vi "2022_day09_Task1_only.vi"() -> ()   [LabVIEW 2021]
panel:
  out "Array 2":bool[][](array[boolean])
  in  "Enum":enum16{"L", "R", "U", "D"}(ring)
  out "Array":cluster{enum16{"L", "R", "U", "D"}, i32}[](array[cluster])
  out "Task 1":i16
  in  "Switch":bool caption="Ex. Data  vs.  User Data"
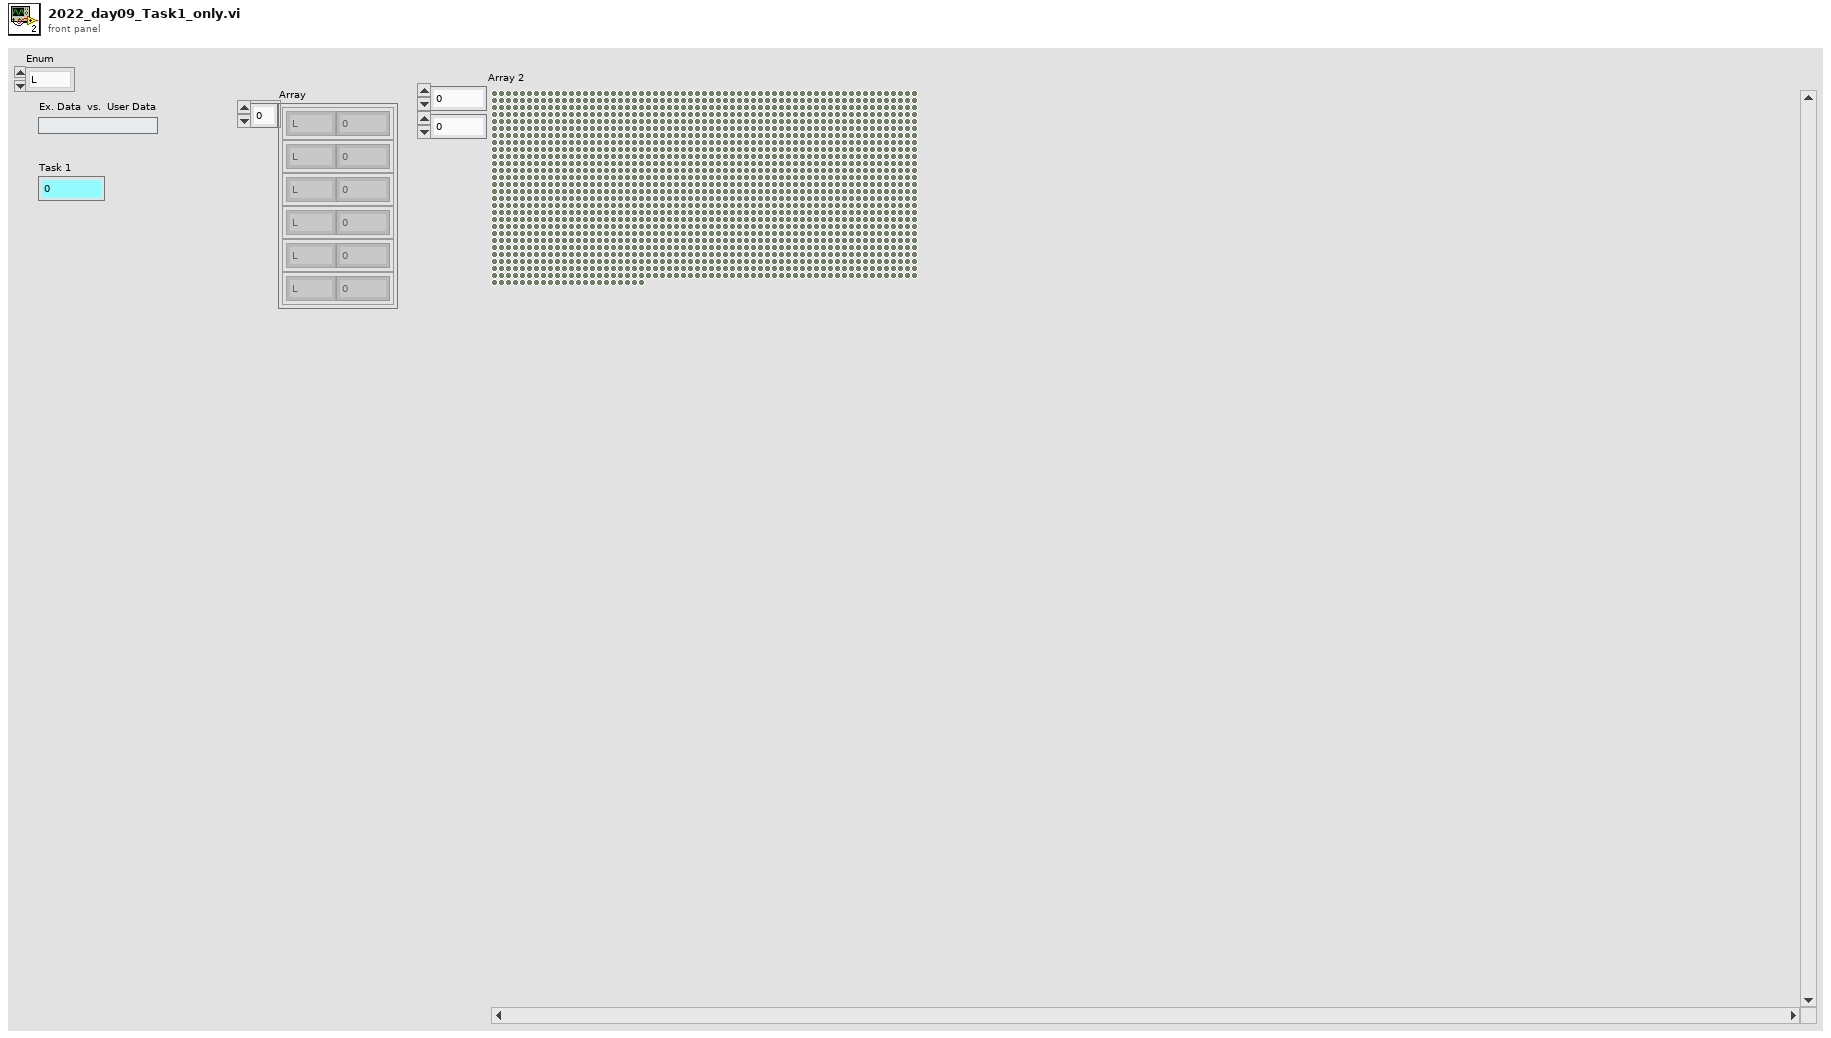
[diagram p1: front panel]
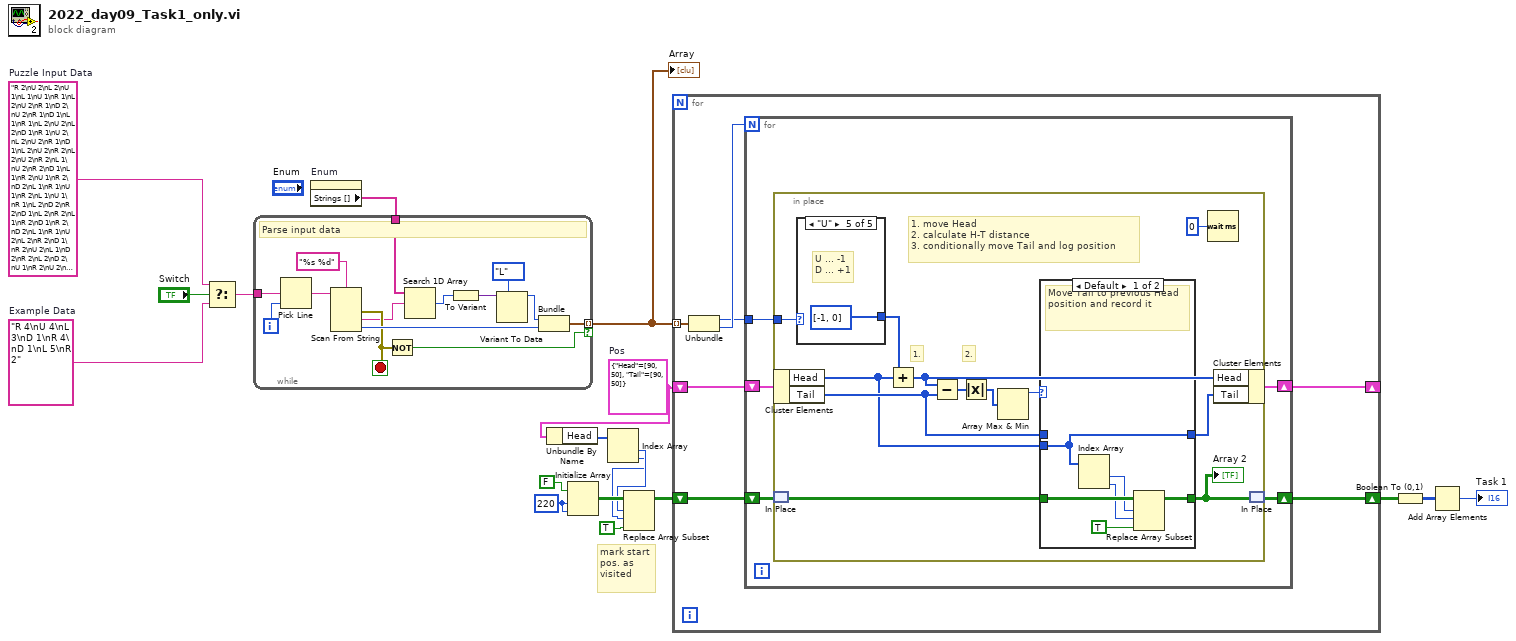
[diagram p0: block diagram]
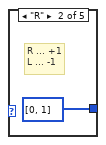
[diagram p4: hidden frame]
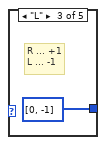
[diagram p5: hidden frame]
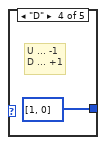
[diagram p6: hidden frame]
diagram:
  w7 = cluster{"Head":i32[], "Tail":i32[]} {"Head"=[90, 50], "Tail"=[90, 50]}  # Pos
  w13 = 220 ("dimension size")
  w17 = "R 2\nU 2\nL 2\nU 1\nL 1\nU 1\nR 1\nL 2\nU 2\nR 1\nD 2\nU 2\nR 1\nD 1\nL 1\nR 1\nL 2\nU 2\nL 2\nD 1\nR 1\nU 2\nL 2\nU 2\nR 1\nD 1\nL 2\nU 2\nR 2\nL 2\nU 2\nR 2\nL 1\nU 2\nR 2\nD 1\nL 1\nR 2\nU 1\nR 2\nD 2\nL 1\nR 1\nU 1\nR 2\nL 1\nU 1\nR 1\nL 2\nD 2\nR 2\nD 1\nL 2\nR 2\nL 1\nR 2\nD 1\nR 2\nD 2\nL 1\nR 1\nU 2\nL 2\nR 2\nD 1\nR 2\nU 2\nL 1\nD 2\nR 2\nL 2\nD 2\nU 1\nR 2\nU 2\nR 2\nD 2\nR 1\nU 2\nD 2\nR 1\nL 1\nR 1\nU 2\nD 2\nR 1\nU 1\nR 1\nL 1\nU 2\nL 2\nD 2\nU 2\nD 2\nR 2\nD 2\nL 1\nU 2\nL 1\nR 1\nD 2\nL 1\nU 1\nD 2\nU 2\nD 2\nR 2\nU 1\nR 1\nU 2\nD 1\nR 2\nD 2\nL 3\nU 1\nD 2\nU 3\nR 3\nL 1\nD 2\nR 1\nD 3\nL 3\nR 1\nD 3\nL 3\nD 1\nR 3\nD 1\nL 1\nD 2\nR 3\nD 1\nU 2\nR 2\nL 1\nD 1\nR 3\nU 2\nL 3\nU 2\nD 2\nR 2\nD 3\nU 1\nD 3\nL 3\nR 2\nL 2\nD 3\nL 2\nU 3\nR 2\nD 1\nR 2\nU 3\nR 3\nU 3\nL 1\nR 3\nD 2\nR 1\nL 3\nR 1\nD 3\nL 3\nD 1\nU 2\nR 3\nU 3\nD 1\nL 2\nR 3\nL 1\nD 2\nL 3\nD 1\nL 3\nD 1\nU 2\nD 3\nR 2\nU 1\nL 3\nR 3\nL 2\nR 1\nL 2\nD 2\nR 3\nU 3\nR 3\nD 2\nU 3\nD 2\nR 3\nD 3\nR 2\nU 1\nL 3\nU 2\nR 2\nL 2\nU 1\nL 3\nD 2\nU 2\nR 1\nL 2\nD 2\nU 3\nR 2\nD 2\nL 3\nU 1\nL 1\nU 2\nR 2\nU 1\nD 2\nU 2\nR 3\nL 1\nU 1\nD 3\nU 4\nL 3\nD 2\nL 3\nU 4\nD 2\nR 4\nL 4\nU 2\nD 3\nU 2\nD 3\nL 3\nU 2\nD 3\nL 1\nU 1\nR 1\nL 4\nR 3\nD 3\nL 2\nU 3\nR 2\nL 1\nU 4\nD 3\nU 1\nL 2\nD 4\nL 1\nR 3\nD 4\nR 1\nL 1\nU 3\nL 3\nD 3\nR 3\nU 1\nL 4\nU 3\nR 3\nL 3\nU 2\nR 3\nL 3\nR 1\nD 3\nR 3\nL 4\nR 3\nD 4\nL 3\nU 2\nR 4\nL 1\nU 1\nR 4\nD 3\nU 1\nR 1\nD 1\nU 3\nR 2\nL 1\nD 1\nL 3\nD 4\nR 4\nU 4\nD 1\nR 3\nD 3\nR 3\nL 4\nR 4\nL 2\nR 2\nD 3\nR 4\nD 2\nU 4\nL 3\nD 1\nR 2\nU 2\nR 3\nD 1\nR 3\nD 1\nL 1\nU 4\nL 2\nU 4\nL 4\nU 3\nR 4\nL 3\nR 3\nL 4\nU 4\nR 4\nD 2\nR 2\nD 3\nU 4\nD 1\nU 1\nD 5\nU 3\nD 5\nU 5\nD 3\nL 3\nU 3\nD 3\nR 1\nD 3\nR 4\nU 4\nD 1\nR 5\nD 5\nR 2\nU 5\nL 2\nU 2\nD 2\nU 4\nR 1\nD 1\nL 2\nR 2\nD 1\nL 5\nR 5\nD 4\nR 5\nL 1\nD 2\nL 3\nU 2\nD 3\nL 1\nR 5\nU 3\nR 1\nD 3\nR 1\nU 1\nR 3\nU 2\nD 5\nL 5\nR 1\nU 3\nL 4\nD 2\nR 1\nD 3\nU 4\nR 3\nL 4\nU 2\nD 3\nU 1\nR 5\nD 3\nL 2\nU 3\nL 5\nU 3\nL 3\nD 5\nL 5\nU 3\nR 2\nD 5\nU 4\nL 5\nU 1\nD 5\nR 3\nD 1\nL 5\nR 2\nD 2\nU 5\nR 1\nD 2\nL 3\nD 2\nL 5\nD 2\nU 5\nL 2\nR 3\nL 3\nD 3\nU 2\nR 5\nL 1\nU 5\nR 5\nL 2\nD 5\nR 3\nL 2\nU 2\nD 3\nR 4\nL 1\nR 3\nD 5\nR 3\nD 4\nR 2\nD 5\nR 3\nL 3\nR 2\nU 2\nL 1\nR 6\nU 6\nL 6\nU 2\nR 6\nD 4\nU 1\nL 1\nR 1\nD 1\nL 6\nD 6\nU 4\nL 6\nD 3\nR 1\nU 1\nD 3\nR 3\nD 5\nU 1\nL 2\nR 6\nU 5\nD 6\nL 6\nR 2\nU 1\nD 1\nL 4\nD 5\nL 6\nU 1\nL 6\nR 5\nU 5\nD 3\nL 5\nR 2\nU 3\nD 1\nL 2\nU 2\nD 1\nL 5\nD 1\nU 5\nR 4\nL 2\nR 5\nD 3\nU 3\nR 2\nU 3\nD 6\nL 5\nR 1\nU 5\nL 1\nR 6\nD 6\nR 6\nL 1\nD 2\nR 5\nL 4\nD 3\nL 5\nR 4\nL 6\nU 1\nL 2\nU 3\nR 4\nD 3\nR 3\nL 1\nD 4\nL 2\nR 5\nD 2\nR 2\nD 5\nU 2\nL 4\nR 4\nU 4\nR 1\nD 3\nL 6\nU 5\nL 5\nD 6\nU 3\nD 6\nR 6\nD 3\nU 6\nL 6\nD 3\nL 6\nR 3\nD 2\nL 4\nD 5\nL 5\nD 2\nL 6\nR 1\nD 1\nL 4\nU 6\nR 1\nL 5\nD 7\nU 2\nR 6\nD 7\nL 2\nR 3\nU 1\nL 3\nR 2\nU 7\nD 7\nU 7\nD 4\nR 2\nL 7\nR 7\nL 5\nR 4\nU 5\nL 5\nU 6\nR 2\nD 3\nL 2\nU 6\nD 5\nR 2\nD 2\nR 5\nU 7\nR 3\nD 1\nL 5\nR 1\nU 3\nD 6\nU 6\nL 7\nU 4\nL 6\nD 1\nL 7\nU 4\nD 7\nL 1\nD 6\nL 2\nR 5\nL 7\nU 3\nD 2\nR 7\nL 2\nU 6\nL 3\nU 6\nL 5\nR 2\nL 7\nD 3\nL 7\nR 1\nL 1\nR 5\nD 6\nL 2\nD 5\nL 4\nD 3\nU 5\nD 1\nR 4\nU 1\nL 2\nR 3\nU 7\nD 6\nU 2\nD 4\nU 5\nD 5\nU 7\nR 2\nD 1\nU 2\nL 2\nU 3\nD 1\nR 4\nD 1\nR 3\nU 1\nR 7\nD 4\nR 3\nD 2\nL 2\nU 4\nL 2\nU 6\nL 4\nD 6\nU 3\nL 1\nU 4\nR 7\nD 6\nL 2\nD 7\nR 4\nU 5\nR 4\nD 5\nR 6\nD 4\nR 4\nU 2\nR 3\nL 7\nR 8\nD 8\nR 5\nU 2\nD 6\nL 2\nR 4\nU 3\nL 1\nR 2\nD 5\nL 1\nD 5\nL 5\nU 1\nR 8\nD 1\nU 1\nL 1\nR 8\nL 3\nR 6\nL 1\nU 3\nR 6\nL 5\nU 2\nL 8\nR 4\nU 4\nR 6\nU 5\nR 1\nL 2\nR 5\nD 1\nU 4\nL 3\nU 3\nR 1\nU 3\nR 8\nL 1\nU 2\nL 7\nD 6\nL 6\nR 4\nD 2\nR 2\nL 8\nD 4\nR 4\nU 4\nL 6\nD 3\nR 7\nD 8\nU 4\nR 4\nU 2\nL 8\nD 5\nL 4\nU 7\nD 8\nU 6\nR 6\nL 5\nD 5\nL 2\nD 1\nR 1\nD 4\nR 5\nL 7\nD 8\nU 2\nD 3\nL 5\nR 4\nL 7\nR 3\nL 1\nD 8\nR 5\nL 8\nR 8\nD 1\nR 4\nD 1\nL 2\nD 5\nL 7\nU 1\nL 4\nR 5\nL 3\nR 9\nD 9\nL 4\nR 6\nL 6\nR 1\nL 3\nR 5\nD 8\nL 1\nU 2\nR 8\nU 7\nD 6\nL 8\nD 1\nL 9\nD 5\nL 1\nD 6\nL 8\nR 2\nL 6\nR 4\nU 1\nR 6\nL 5\nR 5\nL 6\nR 8\nD 5\nL 4\nR 2\nL 7\nR 2\nU 9\nL 6\nR 2\nU 7\nD 4\nU 2\nL 2\nU 8\nR 8\nU 3\nR 6\nD 6\nL 2\nD 4\nL 4\nR 2\nL 1\nU 8\nD 2\nR 2\nL 1\nR 7\nL 8\nD 8\nL 4\nU 4\nR 5\nU 1\nD 8\nL 8\nR 9\nD 6\nL 1\nD 5\nL 9\nU 6\nD 6\nU 3\nD 5\nR 5\nU 9\nL 2\nR 5\nU 9\nL 1\nD 4\nU 4\nL 5\nD 6\nR 3\nL 6\nU 3\nR 4\nU 5\nL 5\nD 8\nL 6\nU 4\nD 1\nU 7\nD 2\nL 3\nR 7\nU 1\nR 4\nU 4\nR 9\nU 3\nD 2\nL 6\nR 9\nU 3\nL 8\nR 10\nU 3\nR 8\nD 8\nL 1\nU 4\nR 5\nU 8\nD 10\nU 10\nL 7\nD 5\nL 2\nR 7\nL 1\nU 10\nR 1\nD 1\nL 5\nR 7\nU 6\nL 3\nR 7\nU 4\nR 3\nU 3\nR 4\nU 8\nL 8\nD 6\nL 5\nU 10\nL 9\nR 3\nU 10\nD 9\nU 5\nD 10\nU 7\nD 6\nU 9\nL 8\nU 3\nD 6\nR 9\nU 9\nD 4\nR 8\nU 7\nR 6\nU 5\nR 5\nU 3\nD 4\nR 9\nL 7\nD 7\nU 1\nL 3\nR 4\nD 8\nL 4\nD 6\nU 1\nR 7\nD 4\nL 9\nD 2\nR 4\nU 10\nD 5\nU 6\nD 6\nR 5\nU 6\nD 6\nL 7\nU 4\nD 1\nL 6\nR 8\nL 7\nU 8\nL 2\nR 6\nL 9\nD 2\nU 9\nD 5\nU 10\nD 1\nR 9\nL 6\nD 7\nU 1\nD 4\nL 3\nR 7\nU 1\nR 6\nD 4\nR 1\nD 4\nL 8\nR 1\nU 10\nD 1\nU 5\nR 6\nU 5\nD 2\nU 10\nR 8\nL 7\nU 6\nL 4\nR 6\nL 7\nU 3\nR 4\nD 1\nL 4\nR 7\nD 2\nL 4\nU 3\nD 6\nU 10\nD 5\nR 8\nU 5\nL 9\nD 4\nL 4\nD 8\nU 9\nR 2\nU 4\nR 4\nU 9\nD 1\nR 7\nU 5\nL 2\nU 10\nR 4\nD 1\nL 3\nR 11\nD 7\nU 7\nD 7\nL 11\nU 2\nD 1\nU 1\nR 1\nU 3\nL 6\nU 10\nL 4\nU 5\nL 10\nD 1\nU 8\nR 7\nL 4\nU 7\nL 9\nU 6\nL 11\nU 3\nR 8\nL 6\nD 9\nL 9\nD 1\nR 7\nL 11\nD 9\nR 7\nU 2\nD 11\nL 4\nD 4\nR 11\nD 7\nU 2\nD 7\nR 2\nD 1\nL 6\nD 11\nR 3\nU 7\nL 10\nU 7\nD 2\nR 2\nU 1\nL 9\nR 11\nL 3\nR 7\nL 2\nD 11\nR 1\nD 4\nR 3\nL 10\nU 5\nD 3\nR 10\nD 8\nU 1\nD 2\nR 10\nL 8\nR 1\nD 8\nU 6\nR 8\nD 8\nL 2\nD 7\nU 4\nL 5\nR 4\nD 4\nU 7\nD 11\nU 11\nR 4\nL 6\nU 3\nL 10\nU 1\nL 11\nU 3\nD 6\nL 11\nR 4\nL 3\nD 12\nL 7\nR 9\nL 9\nU 10\nL 1\nD 6\nL 10\nU 3\nR 6\nD 5\nL 6\nR 8\nD 4\nR 6\nL 6\nD 9\nL 1\nD 11\nU 6\nL 3\nR 10\nU 12\nR 11\nD 10\nU 5\nR 6\nD 12\nU 12\nR 8\nU 5\nD 1\nR 12\nD 1\nR 7\nU 8\nD 5\nU 7\nD 3\nR 7\nD 8\nU 11\nR 2\nU 4\nL 2\nR 1\nL 3\nU 9\nL 5\nD 11\nR 10\nL 3\nU 3\nD 3\nR 1\nL 8\nD 6\nR 7\nU 11\nL 6\nD 1\nR 12\nD 8\nU 7\nR 2\nU 5\nR 4\nU 10\nL 8\nD 5\nU 10\nD 3\nL 6\nR 4\nL 9\nD 6\nR 7\nD 4\nU 10\nD 1\nL 6\nR 1\nL 7\nU 5\nL 9\nU 12\nL 7\nU 6\nD 6\nU 9\nL 7\nU 4\nD 5\nL 1\nU 5\nD 1\nL 10\nD 2\nR 3\nD 13\nU 11\nL 1\nU 1\nD 1\nR 12\nU 13\nL 5\nD 11\nL 9\nU 11\nL 2\nR 6\nD 7\nL 2\nU 5\nR 2\nU 10\nL 9\nD 7\nR 12\nD 10\nL 12\nD 8\nL 8\nR 12\nD 11\nU 12\nL 1\nU 2\nD 6\nR 3\nD 2\nU 9\nL 10\nR 4\nU 2\nD 10\nU 7\nR 6\nU 9\nR 4\nL 3\nU 13\nR 9\nU 6\nD 8\nL 5\nR 11\nL 6\nR 12\nD 5\nU 7\nR 11\nD 1\nL 9\nR 12\nU 2\nR 5\nU 1\nR 9\nU 6\nD 4\nR 2\nU 2\nD 5\nL 9\nR 6\nU 4\nL 6\nR 9\nL 4\nU 3\nL 9\nR 6\nL 5\nD 6\nL 3\nR 6\nL 3\nD 9\nU 5\nD 1\nR 5\nL 3\nU 9\nR 7\nL 8\nR 6\nL 7\nU 4\nD 13\nU 2\nL 1\nU 11\nR 8\nL 13\nD 1\nU 4\nL 13\nD 1\nL 8\nD 13\nL 2\nR 2\nD 1\nL 14\nU 7\nR 11\nL 1\nR 4\nL 5\nR 11\nU 7\nD 8\nL 3\nU 1\nL 12\nU 13\nD 9\nR 1\nL 11\nU 12\nD 5\nU 10\nD 10\nR 9\nL 1\nD 5\nR 7\nL 1\nD 13\nR 10\nU 2\nR 3\nL 14\nD 7\nR 12\nU 13\nL 2\nU 13\nL 3\nU 5\nL 11\nR 8\nD 11\nR 6\nL 11\nR 5\nL 3\nU 1\nL 5\nR 13\nL 12\nD 10\nR 8\nD 6\nL 1\nR 10\nU 5\nR 3\nD 11\nL 8\nR 4\nD 2\nL 1\nR 7\nU 3\nL 14\nR 3\nL 4\nR 13\nL 10\nU 3\nD 1\nL 11\nU 1\nD 6\nR 10\nU 1\nR 2\nL 7\nU 3\nL 5\nU 4\nD 7\nR 8\nU 12\nR 6\nL 2\nD 5\nL 11\nR 4\nL 4\nR 6\nL 3\nR 10\nU 4\nD 9\nU 1\nD 4\nL 12\nD 13\nL 1\nD 6\nR 8\nL 1\nD 9\nL 8\nU 3\nD 3\nU 2\nR 11\nU 10\nL 5\nD 11\nU 12\nD 3\nR 15\nL 1\nR 5\nD 9\nU 15\nD 2\nL 9\nU 9\nD 15\nR 4\nL 9\nR 8\nL 12\nD 5\nR 12\nU 9\nL 9\nU 7\nL 12\nR 11\nU 9\nL 15\nD 9\nL 4\nR 4\nU 13\nD 7\nR 7\nD 8\nU 5\nD 5\nL 15\nD 2\nR 8\nD 10\nR 5\nU 13\nR 1\nL 8\nD 12\nR 2\nL 4\nD 9\nL 9\nD 7\nR 5\nU 15\nR 9\nL 2\nR 8\nU 11\nD 15\nU 13\nD 5\nU 5\nR 11\nU 7\nR 11\nD 12\nU 6\nD 6\nL 8\nD 8\nR 14\nU 13\nR 11\nD 1\nR 4\nU 14\nR 11\nL 8\nD 2\nU 13\nR 15\nL 10\nD 2\nL 3\nR 9\nU 2\nR 8\nU 15\nR 3\nD 4\nL 7\nD 7\nR 1\nD 13\nR 1\nL 13\nU 9\nL 13\nU 10\nL 15\nD 5\nR 11\nD 3\nU 3\nR 4\nL 7\nR 1\nU 13\nR 9\nU 7\nR 10\nD 5\nU 7\nR 6\nL 14\nU 2\nR 8\nD 2\nU 16\nD 12\nR 11\nD 4\nL 8\nU 8\nL 13\nD 5\nR 4\nU 8\nD 15\nR 8\nD 13\nR 16\nU 4\nD 3\nU 5\nD 8\nR 16\nL 13\nU 3\nD 6\nL 9\nR 10\nD 6\nR 16\nD 15\nR 11\nL 8\nD 8\nU 4\nR 16\nD 1\nU 11\nL 15\nR 7\nD 2\nR 1\nD 4\nL 1\nU 15\nD 16\nR 3\nU 10\nD 9\nU 6\nD 15\nR 11\nL 6\nR 2\nU 14\nR 4\nL 15\nR 15\nD 16\nU 9\nD 2\nL 8\nD 15\nR 5\nU 13\nL 15\nD 1\nR 4\nU 14\nD 15\nL 15\nU 13\nR 16\nL 7\nR 4\nD 13\nL 15\nD 3\nL 7\nD 4\nR 12\nD 10\nU 8\nD 6\nL 13\nR 15\nU 12\nL 4\nR 16\nD 1\nR 14\nL 9\nD 13\nU 2\nD 9\nU 16\nL 15\nR 12\nL 14\nR 6\nD 1\nR 2\nL 15\nU 7\nL 16\nU 15\nD 11\nR 11\nL 3\nR 11\nL 15\nU 17\nL 14\nR 4\nU 15\nD 6\nL 2\nR 7\nL 16\nU 4\nL 14\nU 9\nL 7\nD 16\nR 4\nD 2\nR 15\nL 6\nR 6\nD 1\nU 5\nD 14\nU 4\nD 11\nR 5\nU 16\nL 3\nD 7\nR 10\nL 3\nD 8\nL 10\nU 1\nD 16\nL 6\nR 6\nL 14\nR 6\nU 11\nL 17\nD 7\nR 2\nL 12\nD 15\nU 16\nR 2\nU 3\nR 16\nU 12\nL 3\nU 5\nD 1\nR 12\nU 17\nD 11\nL 16\nU 13\nL 5\nD 1\nR 2\nL 10\nU 12\nD 7\nU 6\nR 4\nU 5\nL 3\nR 16\nD 1\nU 14\nR 15\nD 6\nU 14\nR 4\nL 6\nD 11\nR 16\nL 15\nU 7\nL 10\nR 5\nL 15\nR 12\nL 17\nU 5\nD 14\nL 6\nR 2\nU 5\nR 10\nL 8\nD 2\nU 17\nL 13\nD 17\nL 5\nR 11\nL 3\nU 11\nR 1\nL 3\nD 1\nL 7\nD 14\nR 13\nU 9\nD 7\nL 15\nU 5\nD 4\nR 7\nL 10\nD 6\nR 18\nU 5\nR 18\nU 6\nD 17\nU 8\nR 16\nD 12\nR 12\nD 9\nR 9\nU 4\nR 16\nL 1\nD 12\nL 12\nR 11\nD 15\nU 13\nL 8\nR 4\nL 1\nR 1\nD 11\nR 15\nD 3\nL 17\nD 17\nR 11\nU 13\nD 11\nR 4\nD 17\nU 8\nL 1\nD 2\nL 16\nD 6\nL 15\nD 17\nL 8\nU 5\nD 15\nL 15\nU 11\nD 9\nL 18\nU 18\nR 14\nL 4\nU 17\nR 11\nD 18\nU 2\nR 9\nD 15\nR 5\nL 13\nR 2\nL 18\nD 5\nU 14\nL 17\nR 3\nU 4\nR 15\nU 1\nD 15\nU 12\nD 17\nU 11\nL 3\nR 10\nU 13\nR 12\nL 10\nR 1\nD 4\nU 2\nD 14\nR 14\nU 5\nR 16\nU 17\nR 16\nU 18\nR 6\nU 5\nR 18\nU 12\nD 7\nR 9\nL 1\nU 15\nD 10\nL 4\nU 9\nL 3\nU 1\nR 12\nD 14\nU 13\nL 10\nR 8\nU 5\nD 7\nU 1\nL 13\nU 14\nD 18\nL 13\nD 12\nR 2\nL 6\nD 17\nL 18\nR 6\nU 4\nL 7\nR 8\nU 5\nD 1\nL 3\nU 10\nR 5\nD 7\nU 16\nR 12\nU 8\nL 18\nR 1\nL 11\nD 14\nL 19\nR 15\nU 14\nL 8\nR 14\nU 13\nD 18\nU 14\nL 14\nU 11\nL 10\nD 11\nL 11\nR 15\nL 12\nR 10\nL 9\nR 9\nL 9\nD 3\nR 9\nL 6\nR 8\nD 7\nL 18\nD 12\nR 3\nU 7\nR 18\nU 9\nL 14\nD 12\nL 10\nU 15\nL 11\nR 17\nD 7\nR 5\nL 3\nU 13\nD 7\nU 13\nR 16\nD 2\nL 7\nR 15\nL 14\nU 19\nD 3\nL 19\nD 11\nR 8\nD 6\nU 12\nR 5\nU 6\nL 7\nR 4\nL 3\nD 6\nL 17\nU 16\nD 11\nU 12\nD 4\nR 6\nD 10\nL 3\nD 15\nR 5\nL 6\nD 11\nU 17\nL 14\nD 15\nL 1\nD 6\nR 16\nD 11\nU 2\nD 2\nU 7\nD 10\nL 11\nD 19\nL 12\nD 3\nL 18\nU 3"  # Puzzle Input Data
  w15 = "R 4\nU 4\nL 3\nD 1\nR 4\nD 1\nL 5\nR 2"  # Example Data
  # "mark start pos. as visited"
  n1 = Select(t=w17, s="Switch", f=w15) -> (s? t:f=w16:string)
  n2 = property on="Enum" class="Enum (strict)"() -> ("Strings []"=w14:string[])  [unwired: 2 in, 2 out]
  n3 = while {
    tunnel: w16 -> [w27]
    tunnel: [w28] -> w11 mode=indexing if=w31
    tunnel: w14 -> [w24]
    i -> [w32]
    stop <- w25 stop-if-true
    # "Parse input data"
    n4 = Pick Line(multi-line string=w27, line index=w32) -> (output string=w26:string)  [unwired: 1 in]
    n5 = Scan From String(format string="%s %d", input string=w26) -> (error out=w25:errorcluster, output 1=w23:string, output 2=w29:i32)  [unwired: 4 in, 2 out]
    n6 = Not(x=w25) -> (.not. x?=w31:bool)
    n7 = Search 1D Array(1D array=w24, element=w23) -> (index of element=w20:i32)  [unwired: 1 in]
    n8 = To Variant(anything=w20) -> (Variant=w22:variant)
    n9 = Variant To Data(type=enum16{"L", "R", "U", "D"}."L", Variant=w22) -> (data=w19:enum16{"L", "R", "U", "D"})  [unwired: 1 in, 1 out]
    n10 = Bundle(w19, w29) -> (w28:cluster{enum16{"L", "R", "U", "D"}, i32})  [unwired: 1 in]
  }
  "Array" <- w11
  n11 = Unbundle By Name(w7) -> ("Head"=w6:i32[])
  n12 = Initialize Array(FALSE, w13, w13) -> (w9:bool[][])
  n13 = Index Array(array=w6) -> (element #1=w5:i32, element #2=w4:i32)  [unwired: 2 in]
  n14 = Replace Array Subset(array=w9, new element=TRUE ("new element/subarray"), index (row)=w5, index (col)=w4) -> (w8:bool[][])
  n15 = for {
    tunnel: w11 -> [w39] mode=indexing
    shift-right: [w33] -> w3
    shift-left: w8 -> [w34]
    shift-right: [w35] -> _
    shift-left: w7 -> [w36]
    n16 = Unbundle(w39) -> (w37:enum16{"L", "R", "U", "D"}, w38:i32)
    n17 = for {
      N: w38 -> [_]
      tunnel: w37 -> [w44]
      shift-right: [w42] -> w35
      shift-left: w36 -> [w43]
      shift-right: [w40] -> w33
      shift-left: w34 -> [w41]
      n18 = in-place {
        in-place-border: w44 -> [w56]
        # "2."
        # "1. move Head\n2. calculate H-T distance\n3. conditionally move Tail and log position"
        # "1."
        n19 = in-place-cluster #1(w43) -> ("Head"=w48:i32[], "Tail"=w50:i32[])
        n20 = in-place-match #2(w41) -> (w47:bool[][])
        n21 = case shown="\"U\"" w56 {
          tunnel: [_ i32[] [0, 1] ("Move") i32[] [0, -1] ("Move") i32[] [1, 0] ("Move") i32[] [-1, 0] ("Move")] -> w55
          frame Default {
            # "this should not happen"
          }
          frame "R" {
            # "R ... +1\nL ... -1"
          }
          frame "L" {
            # "R ... +1\nL ... -1"
          }
          frame "D" {
            # "U ... -1\nD ... +1"
          }
          frame "U" {
            # "U ... -1\nD ... +1"
          }
        }
        n22 = Add(x=w55, y=w48) -> (x+y=w54:i32[])
        n23 = Subtract(x=w54, y=w50) -> (x-y=w53:i32[])
        n24 = Absolute Value(x=w53) -> (abs(x)=w52:i32[])
        n25 = Array Max & Min(array=w52) -> (max value=w51:i32)  [unwired: 3 out]
        n26 = case shown="Default" w51 {
          tunnel: w50 -> [_ w64]
          tunnel: [w60 w64] -> w49
          tunnel: w48 -> [w60 _]
          tunnel: w47 -> [w62 w63]
          tunnel: [w61 w63] -> w45
          frame Default {
            # "Move Tail to previous Head position and record it"
            n27 = Index Array(array=w60) -> (element #1=w59:i32, element #2=w58:i32)  [unwired: 2 in]
            n28 = Replace Array Subset(array=w62, new element=TRUE ("new element/subarray"), index (row)=w59, index (col)=w58) -> (w61:bool[][])
          }
          frame 0, 1 {
            # "T-H distance is 1 don't move Tail"
          }
        }
        "Array 2" <- w45
        n29 = Wait (ms)(milliseconds to wait=u32 0) -> ()  [unwired: 1 out]
        n30 = in-place-cluster #1("Head"=w54, "Tail"=w49) -> (w42:cluster{"Head":i32[], "Tail":i32[]})
        n31 = in-place-match #2(w45) -> (w40:bool[][])
      }
    }
  }
  n32 = Boolean To (0,1)(Boolean=w3) -> (0, 1=w2:i16[][])
  n33 = Add Array Elements(numeric array=w2) -> (sum=→"Task 1":i16)
